vi "Add Target Listener.vi"(8 "error in":errorcluster, 10 "queue out":T2, 11 "VisionServerRef in":T1) -> (0 "error out":errorcluster, 3 "VisionServerRef out":T1)   [LabVIEW 2016, in "Vision Server.lvclass"]
uses:
  Vision Server.lvclass
  typedef/Target Listener Queue.ctl
  typedef/Target Message Processed.ctl
  typedef/Target Vector.ctl
  typedef/Vision Server Ref.ctl
  Vision Server.lvclass/Vision Server.ctl
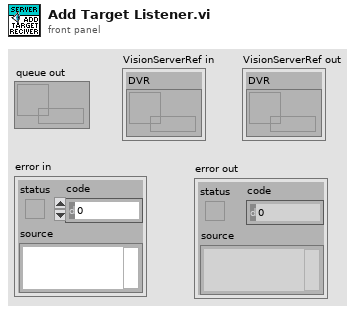
[diagram p1: front panel]
types:
  T1 = typedef "Vision Server.lvclass/Vision Server Ref.ctl" = cluster{"DVR":refnum<data-value>}
  T2 = typedef "Vision Server.lvclass/Target Listener Queue.ctl" = refnum<queue>
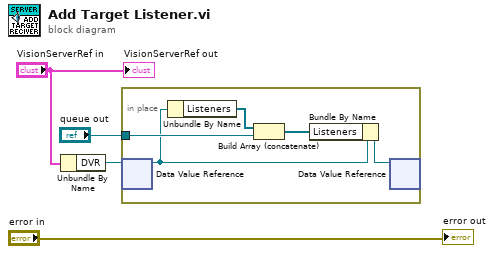
[diagram p0: block diagram]
diagram:
  n1 = Unbundle By Name("VisionServerRef in") -> ("DVR"=w1:refnum<data-value>)
  n2 = in-place {
    in-place-border: "queue out" -> [w8]
    n3 = in-place-dvr #1(w1) -> (w7:refnum<class "Vision Server.lvclass">)  [unwired: 1 out]
    n4 = Unbundle By Name(w7) -> ("Listeners"=w9:T2[])
    n5 = Build Array (concatenate)(w9, w8) -> (w6:T2[])
    n6 = Bundle By Name(cluster=w7, "Listeners"=w6) -> (w5:refnum<class "Vision Server.lvclass">)
    n7 = in-place-dvr #1(w5) -> ()  [unwired: 2 out]
  }
  "error out" <- "error in"
  "VisionServerRef out" <- "VisionServerRef in"
